vi "Get K Coeff.vi"(7 "K Coeff":T1, 10 "Number of Trials/Parts":i32, 11 "G":i32) -> (3 "K Coeff":dbl)   [LabVIEW 2018, in "GRR Core.lvclass"]
uses:
  GRR Core.lvclass
  Typedefs/K Coeff.ctl
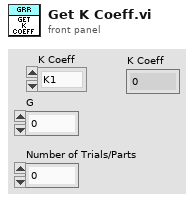
[diagram p1: front panel]
types:
  T1 = typedef "GRR Core.lvclass/K Coeff.ctl" = enum16{"K1", "K2 or K3"}
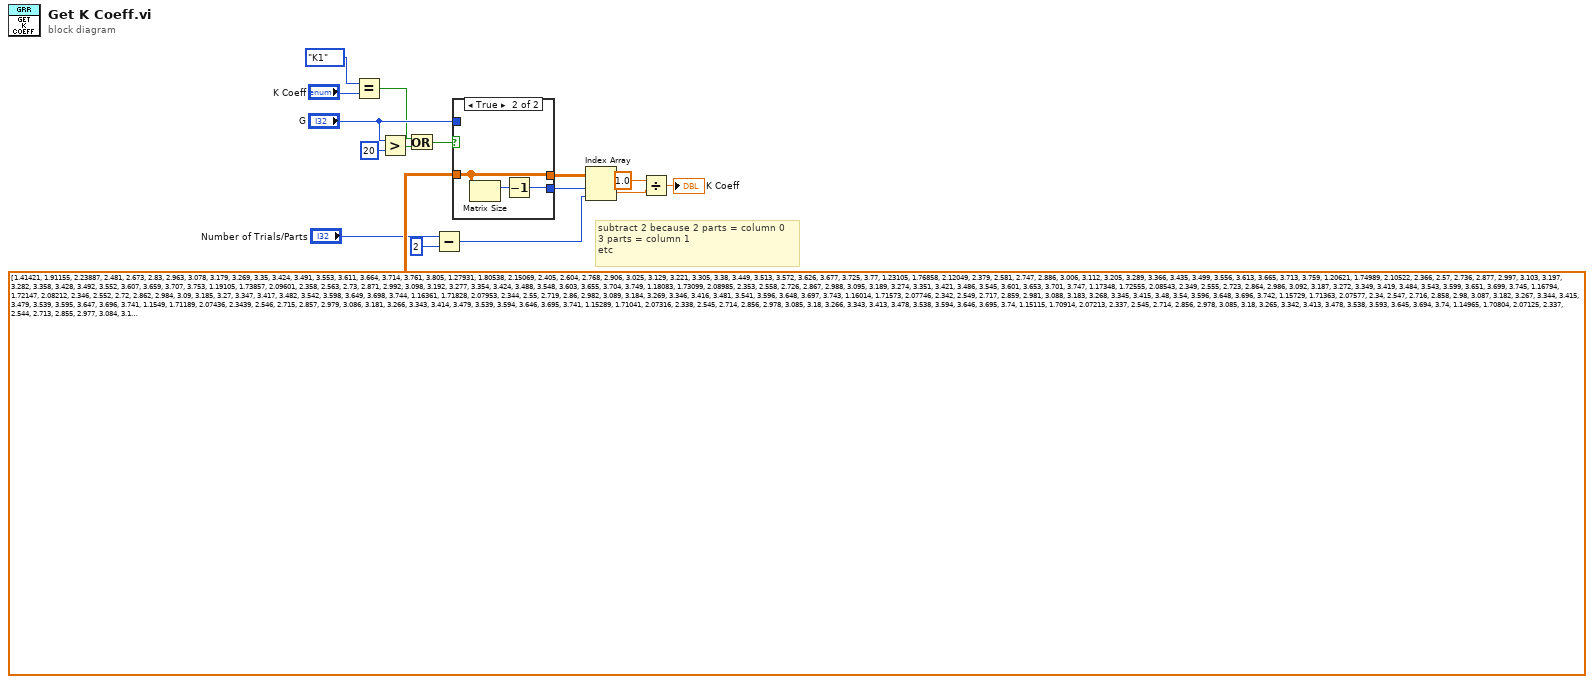
[diagram p0: block diagram]
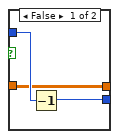
[diagram p2: hidden frame]
diagram:
  # "subtract 2 because 2 parts = column 0\n3 parts = column 1\netc"
  n1 = Equal?(x=K_Coeff."K1" ("K Coeff"), y="K Coeff") -> (x = y?=w13:bool)
  n2 = Greater?(x="G", y=20) -> (0:w14:bool)
  n3 = Or(x=w13, y=w14) -> (x .or. y?=w12:bool)
  n4 = Subtract(x="Number of Trials/Parts", y=2) -> (x-y=w6:i32)
  n5 = case shown="True" w12 {
    tunnel: dbl[][] [[1.41421, 1.91155, 2.23887, 2.481, 2.673, 2.83, 2.963, 3.078, 3.179, 3.269, 3.35, 3.424, 3.491, 3.553, 3.611, 3.664, 3.714, 3.761, 3.805], [1.27931, 1.80538, 2.15069, 2.405, 2.604, 2.768, 2.906, 3.025, 3.129, 3.221, 3.305, 3.38, 3.449, 3.513, 3.572, 3.626, 3.677, 3.725, 3.77], [1.23105, 1.76858, 2.12049, 2.379, 2.581, 2.747, 2.886, 3.006, 3.112, 3.205, 3.289, 3.366, 3.435, 3.499, 3.556, 3.613, 3.665, 3.713, 3.759], [1.20621, 1.74989, 2.10522, 2.366, 2.57, 2.736, 2.877, 2.997, 3.103, 3.197, 3.282, 3.358, 3.428, 3.492, 3.552, 3.607, 3.659, 3.707, 3.753], [1.19105, 1.73857, 2.09601, 2.358, 2.563, 2.73, 2.871, 2.992, 3.098, 3.192, 3.277, 3.354, 3.424, 3.488, 3.548, 3.603, 3.655, 3.704, 3.749], [1.18083, 1.73099, 2.08985, 2.353, 2.558, 2.726, 2.867, 2.988, 3.095, 3.189, 3.274, 3.351, 3.421, 3.486, 3.545, 3.601, 3.653, 3.701, 3.747], [1.17348, 1.72555, 2.08543, 2.349, 2.555, 2.723, 2.864, 2.986, 3.092, 3.187, 3.272, 3.349, 3.419, 3.484, 3.543, 3.599, 3.651, 3.699, 3.745], [1.16794, 1.72147, 2.08212, 2.346, 2.552, 2.72, 2.862, 2.984, 3.09, 3.185, 3.27, 3.347, 3.417, 3.482, 3.542, 3.598, 3.649, 3.698, 3.744], [1.16361, 1.71828, 2.07953, 2.344, 2.55, 2.719, 2.86, 2.982, 3.089, 3.184, 3.269, 3.346, 3.416, 3.481, 3.541, 3.596, 3.648, 3.697, 3.743], [1.16014, 1.71573, 2.07746, 2.342, 2.549, 2.717, 2.859, 2.981, 3.088, 3.183, 3.268, 3.345, 3.415, 3.48, 3.54, 3.596, 3.648, 3.696, 3.742], [1.15729, 1.71363, 2.07577, 2.34, 2.547, 2.716, 2.858, 2.98, 3.087, 3.182, 3.267, 3.344, 3.415, 3.479, 3.539, 3.595, 3.647, 3.696, 3.741], [1.1549, 1.71189, 2.07436, 2.3439, 2.546, 2.715, 2.857, 2.979, 3.086, 3.181, 3.266, 3.343, 3.414, 3.479, 3.539, 3.594, 3.646, 3.695, 3.741], [1.15289, 1.71041, 2.07316, 2.338, 2.545, 2.714, 2.856, 2.978, 3.085, 3.18, 3.266, 3.343, 3.413, 3.478, 3.538, 3.594, 3.646, 3.695, 3.74], [1.15115, 1.70914, 2.07213, 2.337, 2.545, 2.714, 2.856, 2.978, 3.085, 3.18, 3.265, 3.342, 3.413, 3.478, 3.538, 3.593, 3.645, 3.694, 3.74], [1.14965, 1.70804, 2.07125, 2.337, 2.544, 2.713, 2.855, 2.977, 3.084, 3.179, 3.265, 3.342, 3.412, 3.477, 3.537, 3.593, 3.645, 3.694, 3.74], [1.14833, 1.70708, 2.07047, 2.336, 2.543, 2.712, 2.846, 2.977, 3.084, 3.179, 3.264, 3.342, 3.412, 3.477, 3.537, 3.593, 3.665, 3.693, 3.739], [1.14717, 1.70623, 2.06978, 2.335, 2.543, 2.712, 2.854, 2.976, 3.084, 3.179, 3.264, 3.341, 3.412, 3.477, 3.537, 3.592, 3.644, 3.693, 3.74], [1.14613, 1.70547, 2.06917, 2.542, 2.711, 2.854, 2.976, 3.083, 3.083, 3.179, 3.263, 3.341, 3.412, 3.477, 3.536, 3.592, 3.644, 3.693, 3.734], [1.1452, 1.7048, 2.06862, 2.334, 2.542, 2.711, 2.853, 2.976, 3.083, 3.178, 3.263, 3.341, 3.411, 3.476, 3.536, 3.592, 3.644, 3.693, 3.739], [1.14437, 1.70419, 2.06813, 2.334, 2.541, 2.711, 2.853, 2.976, 3.083, 3.178, 3.263, 3.34, 3.411, 3.476, 3.536, 3.592, 3.644, 3.963, 3.739], [1.128, 1.693, 2.059, 2.326, 2.534, 2.704, 2.847, 2.97, 3.078, 3.173, 3.259, 3.336, 3.407, 3.472, 3.532, 3.588, 3.64, 3.689, 3.735]] ("all rows") -> [w18 w21]
    tunnel: "G" -> [w19 _]
    tunnel: [w18 w21] -> w11
    tunnel: [w17 w20] -> w10
    frame False {
      n6 = Decrement(x=w19) -> (x-1=w17:i32)
    }
    frame True {
      n7 = Matrix Size(0:w21) -> (1:w22:i32)  [unwired: 1 out]
      n8 = Decrement(x=w22) -> (x-1=w20:i32)
    }
  }
  n9 = Index Array(array=w11, index (row)=w10, index (col)=w6) -> (element=w5:dbl)
  n10 = Divide(x=1.0, y=w5) -> (x/y=→"K Coeff":dbl)
